vi "sub_create_error_from_http_code.vi"(8 "error in (no error)":errorcluster, 9 "Error String":string, 10 "HTTP Code":i32) -> (0 "error out":errorcluster, 2 "connected":bool)   [LabVIEW 2013, in "daqio minimal.lvlib"]
doc: "This VI will return a custom error from an http error code."
uses:
  daqio minimal.lvlib
  <vilib>/Utility/error.llb/DialogType.ctl
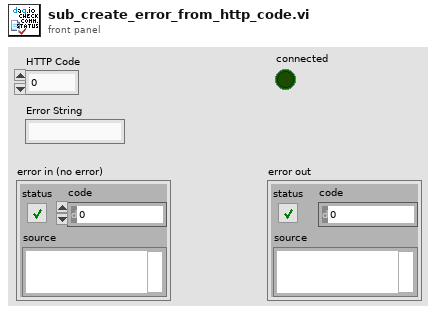
[diagram p1: front panel]
types:
  T1 = typedef "DialogType.ctl" = u16
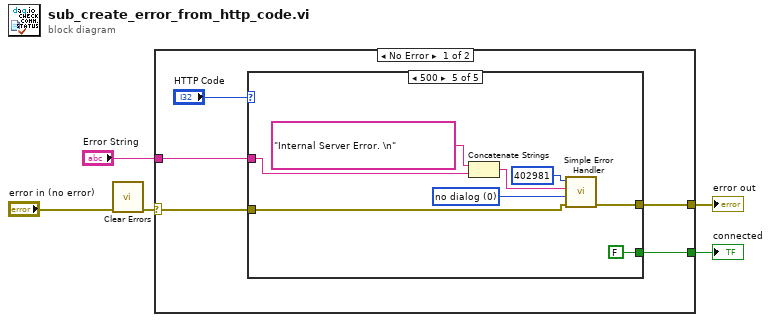
[diagram p0: block diagram]
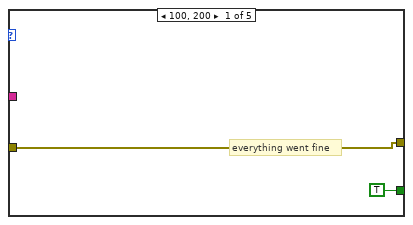
[diagram p2: hidden frame]
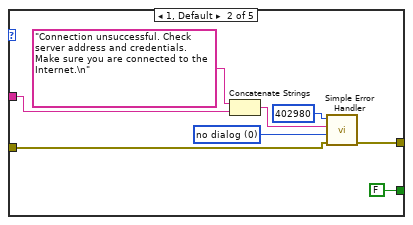
[diagram p3: hidden frame]
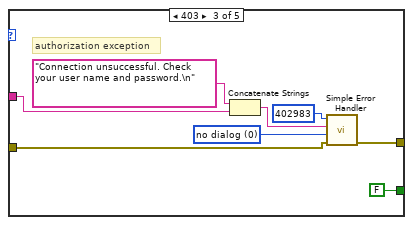
[diagram p4: hidden frame]
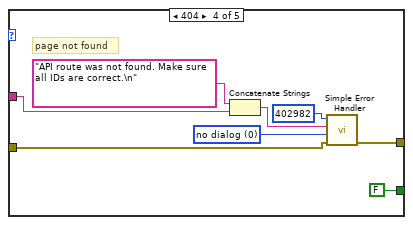
[diagram p5: hidden frame]
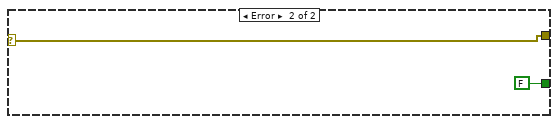
[diagram p6: hidden frame]
diagram:
  n1 = call <vilib>:"Clear Errors.vi"("error in (no error)"="error in (no error)") -> ("error out"=w2:errorcluster)  [unwired: 6 in]
  n2 = case shown="No Error" w2 {
    selector: w2 -> [w7 w46]
    tunnel: [w9 w46] -> w5
    tunnel: [w10 FALSE] -> w4
    tunnel: "Error String" -> [w6 _]
    frame No Error {
      n3 = case shown="500" "HTTP Code" {
        tunnel: [w11 w20 w26 w35 w41] -> w9
        tunnel: [TRUE FALSE FALSE FALSE FALSE] -> w10
        tunnel: w7 -> [w11 w17 w25 w33 w42]
        tunnel: w6 -> [_ w13 w22 w31 w37]
        frame 100, 200 {
          # "everything went fine"
        }
        frame 1, Default {
          w19 = T1 0 items=["no dialog", "OK message", "continue or stop message", "OK message + warnings", "continue/stop + warnings"] ("type of dialog (OK msg:1)")
          n4 = Concatenate Strings("Connection unsuccessful. Check server address and credentials. Make sure you are connected to the Internet.\n" ("error source (\" \")"), w13) -> (w14:string)
          n5 = call <vilib>:"Simple Error Handler.vi"("error code (no error:0)"=402980, "error source (\" \")"=w14, "type of dialog (OK msg:1)"=w19, "error in (no error)"=w17) -> ("error out"=w20:errorcluster)  [unwired: 1 in, 4 out]
        }
        frame 403 {
          w27 = T1 0 items=["no dialog", "OK message", "continue or stop message", "OK message + warnings", "continue/stop + warnings"] ("type of dialog (OK msg:1)")
          # "authorization exception"
          n6 = Concatenate Strings("Connection unsuccessful. Check your user name and password.\n" ("error source (\" \")"), w22) -> (w21:string)
          n7 = call <vilib>:"Simple Error Handler.vi"("error code (no error:0)"=402983, "error source (\" \")"=w21, "type of dialog (OK msg:1)"=w27, "error in (no error)"=w25) -> ("error out"=w26:errorcluster)  [unwired: 1 in, 4 out]
        }
        frame 404 {
          w34 = T1 0 items=["no dialog", "OK message", "continue or stop message", "OK message + warnings", "continue/stop + warnings"] ("type of dialog (OK msg:1)")
          # "page not found"
          n8 = Concatenate Strings("API route was not found. Make sure all IDs are correct.\n" ("error source (\" \")"), w31) -> (w29:string)
          n9 = call <vilib>:"Simple Error Handler.vi"("error code (no error:0)"=402982, "error source (\" \")"=w29, "type of dialog (OK msg:1)"=w34, "error in (no error)"=w33) -> ("error out"=w35:errorcluster)  [unwired: 1 in, 4 out]
        }
        frame 500 {
          w43 = T1 0 items=["no dialog", "OK message", "continue or stop message", "OK message + warnings", "continue/stop + warnings"] ("type of dialog (OK msg:1)")
          n10 = Concatenate Strings("Internal Server Error. \n" ("error source (\" \")"), w37) -> (w39:string)
          n11 = call <vilib>:"Simple Error Handler.vi"("error code (no error:0)"=402981, "error source (\" \")"=w39, "type of dialog (OK msg:1)"=w43, "error in (no error)"=w42) -> ("error out"=w41:errorcluster)  [unwired: 1 in, 4 out]
        }
      }
    }
    frame Error {
    }
  }
  "error out" <- w5
  "connected" <- w4
